vi "StackTypedef.vi"(11 "StackArray":T1(array[cluster])) -> (2 "Value String":string, 3 "Boolean":bool)   [LabVIEW 2021]
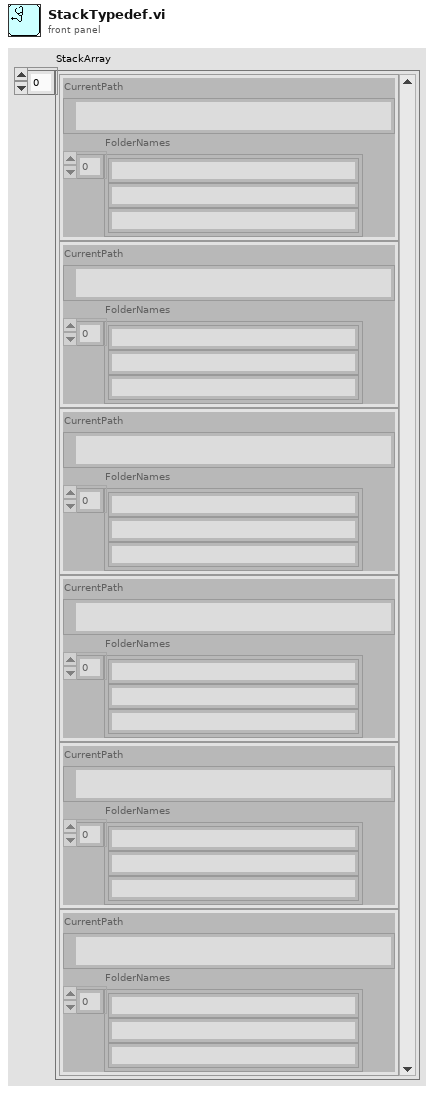
[diagram p1: front panel]
types:
  T1 = cluster{"CurrentPath":path, "FolderNames":string[]}[]
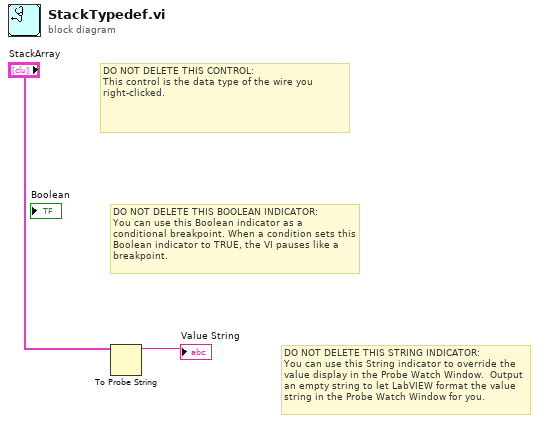
[diagram p0: block diagram]
diagram:
  # "DO NOT DELETE THIS STRING INDICATOR: \nYou can use this String indicator to override the value display in the Probe Watch Window.  Output an empty string to let LabVIEW format the value string in the Probe Watch Window for you."
  # "DO NOT DELETE THIS BOOLEAN INDICATOR: \nYou can use this Boolean indicator as a conditional breakpoint. When a condition sets this Boolean indicator to TRUE, the VI pauses like a breakpoint."
  # "DO NOT DELETE THIS CONTROL: \nThis control is the data type of the wire you right-clicked."
  n1 = To Probe String(7:"StackArray") -> (3:→"Value String":string)  [unwired: 2 in, 1 out]
